vi "Convert C to F.vi"(11 "Celcius":dbl) -> (3 "Farenheit":dbl)   [LabVIEW 2019]
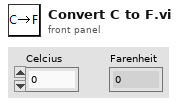
[diagram p1: front panel]
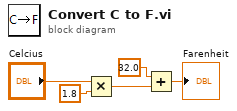
[diagram p0: block diagram]
diagram:
  n1 = Multiply(x="Celcius", y=1.8) -> (x*y=w4:dbl)
  n2 = Add(x=32.0, y=w4) -> (x+y=→"Farenheit":dbl)
